vi "Unscale(Table).vi"(9 "coercion":T1, 10 "scales":T2[](array[typedef]), 11 "scale value":dbl format="%#_13g") -> (3 "unscale value":dbl)   [LabVIEW 2015, in "Scale.lvlib"]
uses:
  Scale.lvlib
  ScaleMapping.ctl
  Coercion.ctl
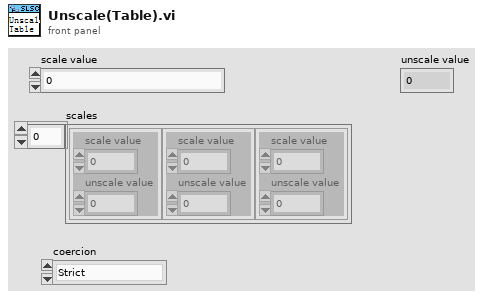
[diagram p1: front panel]
types:
  T1 = typedef "Scale.lvlib/Coercion.ctl" = enum16{"Strict", "RoundToNearest", "Interpolate"}
  T2 = typedef "Scale.lvlib/ScaleMapping.ctl" = cluster{"scale value":dbl, "unscale value":dbl}
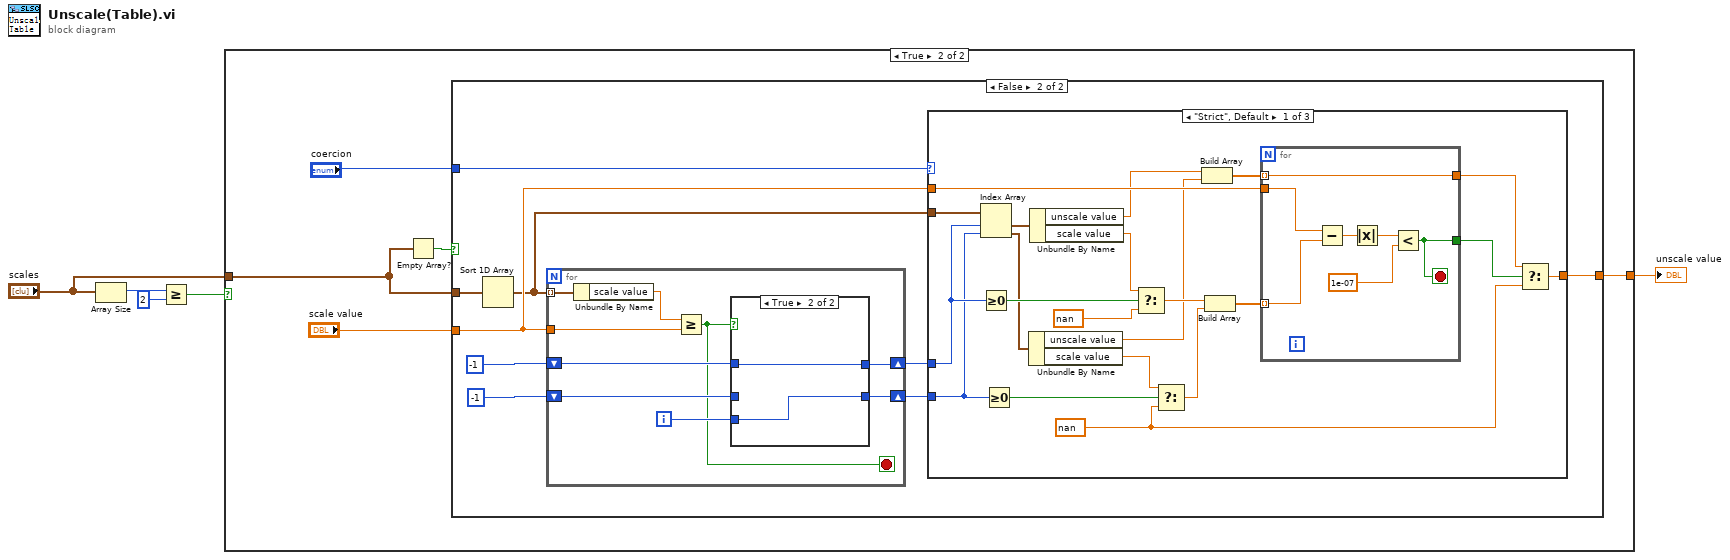
[diagram p0: block diagram]
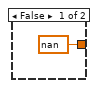
[diagram p2: hidden frame]
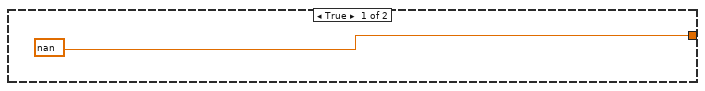
[diagram p3: hidden frame]
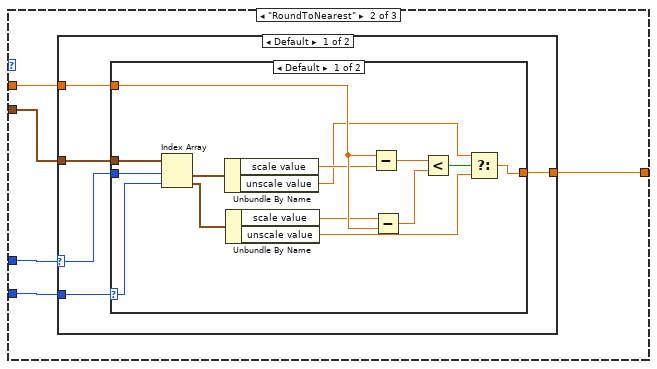
[diagram p4: hidden frame]
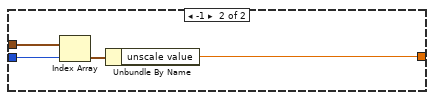
[diagram p5: hidden frame]
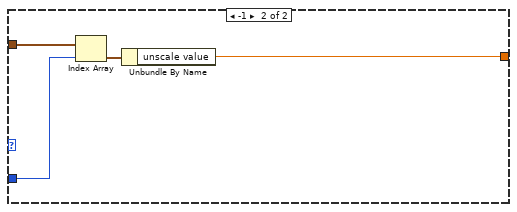
[diagram p6: hidden frame]
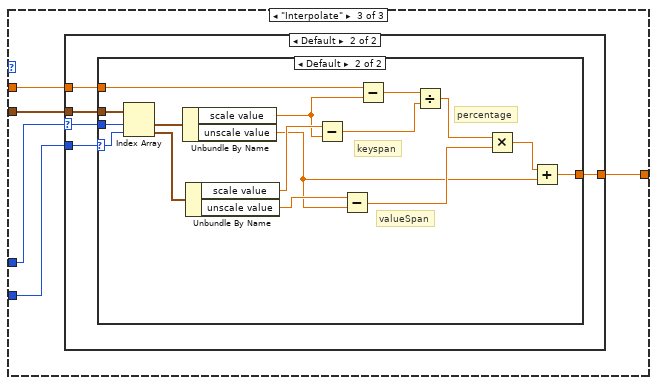
[diagram p7: hidden frame]
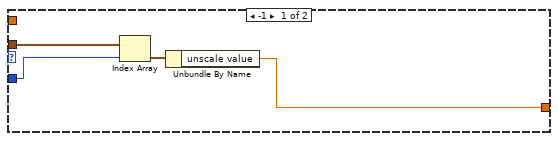
[diagram p8: hidden frame]
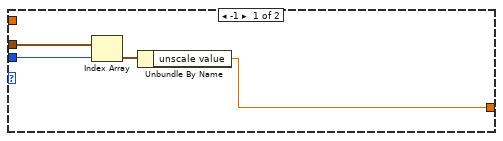
[diagram p9: hidden frame]
diagram:
  n1 = Array Size(array="scales") -> (size(s)=w5:i32)
  n2 = Greater Or Equal?(x=w5, y=2) -> (x >= y?=w3:bool)
  n3 = case shown="True" w3 {
    tunnel: "scales" -> [_ w9]
    tunnel: [nan ("unscale value") w8] -> w2
    frame False {
    }
    frame True {
      n4 = Empty Array?(array=w9) -> (empty?=w10:bool)
      n5 = case shown="False" w10 {
        tunnel: w9 -> [_ w16]
        tunnel: "coercion" -> [_ w19]
        tunnel: "scale value" -> [_ w15]
        tunnel: [nan ("f") w14] -> w8
        frame True {
        }
        frame False {
          n6 = Sort 1D Array(array=w16) -> (sorted array=w13:T2[])
          n7 = for {
            tunnel: w13 -> [w124] mode=indexing
            tunnel: w15 -> [w122]
            shift-right: [w119] -> w18
            shift-left: -1 -> [w118]
            shift-right: [w120] -> w17
            shift-left: -1 -> [w117]
            i -> [w121]
            stop <- w116 stop-if-true
            n8 = Unbundle By Name(w124) -> ("scale value"=w123:dbl)
            n9 = Greater Or Equal?(x=w123, y=w122) -> (x >= y?=w116:bool)
            n10 = case shown="True" w116 {
              tunnel: w121 -> [w125 w128]
              tunnel: [w126 w128] -> w120
              tunnel: [w125 w127] -> w119
              tunnel: w118 -> [_ w127]
              tunnel: w117 -> [w126 _]
              frame False {
              }
              frame True {
              }
            }
          }
          n11 = case shown="\"Strict\", Default" w19 {
            tunnel: w18 -> [w41 w54 w82]
            tunnel: w17 -> [w38 w52 w85]
            tunnel: w13 -> [w27 w53 w86]
            tunnel: w15 -> [w30 w50 w84]
            tunnel: [w28 w51 w83] -> w14
            frame "Strict", Default {
              w22 = nan
              n12 = Index Array(array=w27, index #1=w41, index #2=w38) -> (element #1=w40:T2, element #2=w37:T2)
              n13 = Greater Or Equal To 0?(x=w41) -> (x >= 0?=w42:bool)
              n14 = Greater Or Equal To 0?(x=w38) -> (x >= 0?=w35:bool)
              n15 = Unbundle By Name(w37) -> ("unscale value"=w23:dbl, "scale value"=w36:dbl)
              n16 = Unbundle By Name(w40) -> ("unscale value"=w24:dbl, "scale value"=w39:dbl)
              n17 = Select(t=w39, s=w42, f=nan) -> (s? t:f=w33:dbl)
              n18 = Select(t=w36, s=w35, f=w22) -> (s? t:f=w32:dbl)
              n19 = Build Array(w24, w23) -> (w26:dbl[])
              n20 = Build Array(w33, w32) -> (w31:dbl[])
              n21 = for {
                tunnel: w31 -> [w48] mode=indexing
                tunnel: w30 -> [w49]
                tunnel: [w45] -> w29
                tunnel: w26 -> [w43] mode=indexing
                tunnel: [w43] -> w25
                stop <- w45 stop-if-true
                n22 = Subtract(x=w49, y=w48) -> (x-y=w47:dbl)
                n23 = Absolute Value(x=w47) -> (abs(x)=w44:dbl)
                n24 = Less?(x=w44, y=1e-07) -> (x < y?=w45:bool)
              }
              n25 = Select(t=w25, s=w29, f=w22) -> (s? t:f=w28:dbl)
            }
            frame "RoundToNearest" {
              n26 = case shown="Default" w54 {
                selector: w54 -> [w57 _]
                tunnel: w53 -> [w58 w78]
                tunnel: w52 -> [w59 w81]
                tunnel: [w56 w79] -> w51
                tunnel: w50 -> [w55 _]
                frame Default {
                  n27 = case shown="Default" w59 {
                    selector: w59 -> [w71 _]
                    tunnel: w58 -> [w73 w76]
                    tunnel: w57 -> [w72 w75]
                    tunnel: [w63 w74] -> w56
                    tunnel: w55 -> [w69 _]
                    frame Default {
                      n28 = Index Array(array=w73, index #1=w72, index #2=w71) -> (element #1=w70:T2, element #2=w62:T2)
                      n29 = Unbundle By Name(w70) -> ("scale value"=w65:dbl, "unscale value"=w61:dbl)
                      n30 = Unbundle By Name(w62) -> ("scale value"=w64:dbl, "unscale value"=w60:dbl)
                      n31 = Subtract(x=w69, y=w65) -> (x-y=w68:dbl)
                      n32 = Subtract(x=w64, y=w69) -> (x-y=w67:dbl)
                      n33 = Less?(x=w68, y=w67) -> (x < y?=w66:bool)
                      n34 = Select(t=w61, s=w66, f=w60) -> (s? t:f=w63:dbl)
                    }
                    frame -1 {
                      n35 = Index Array(array=w76, index=w75) -> (element=w77:T2)
                      n36 = Unbundle By Name(w77) -> ("unscale value"=w74:dbl)
                    }
                  }
                }
                frame -1 {
                  n37 = Index Array(array=w78, index=w81) -> (element=w80:T2)
                  n38 = Unbundle By Name(w80) -> ("unscale value"=w79:dbl)
                }
              }
            }
            frame "Interpolate" {
              n39 = case shown="Default" w82 {
                selector: w82 -> [_ w92]
                tunnel: w86 -> [w90 w95]
                tunnel: w85 -> [w89 w91]
                tunnel: w84 -> [_ w94]
                tunnel: [w87 w93] -> w83
                frame -1 {
                  n40 = Index Array(array=w90, index=w89) -> (element=w88:T2)
                  n41 = Unbundle By Name(w88) -> ("unscale value"=w87:dbl)
                }
                frame Default {
                  n42 = case shown="Default" w91 {
                    selector: w91 -> [_ w104]
                    tunnel: w95 -> [w98 w115]
                    tunnel: w94 -> [_ w113]
                    tunnel: [w96 w107] -> w93
                    tunnel: w92 -> [w97 w106]
                    frame -1 {
                      n43 = Index Array(array=w98, index=w97) -> (element=w99:T2)
                      n44 = Unbundle By Name(w99) -> ("unscale value"=w96:dbl)
                    }
                    frame Default {
                      # "percentage"
                      # "keyspan"
                      # "valueSpan"
                      n45 = Index Array(array=w115, index #1=w106, index #2=w104) -> (element #1=w114:T2, element #2=w105:T2)
                      n46 = Unbundle By Name(w114) -> ("scale value"=w102:dbl, "unscale value"=w100:dbl)
                      n47 = Unbundle By Name(w105) -> ("scale value"=w103:dbl, "unscale value"=w101:dbl)
                      n48 = Subtract(x=w103, y=w102) -> (x-y=w109:dbl)
                      n49 = Subtract(x=w101, y=w100) -> (x-y=w110:dbl)
                      n50 = Subtract(x=w113, y=w102) -> (x-y=w112:dbl)
                      n51 = Divide(x=w112, y=w109) -> (x/y=w111:dbl)
                      n52 = Multiply(x=w111, y=w110) -> (x*y=w108:dbl)
                      n53 = Add(x=w108, y=w100) -> (x+y=w107:dbl)
                    }
                  }
                }
              }
            }
          }
        }
      }
    }
  }
  "unscale value" <- w2
